vi "Connect_Netpie.vi"(6 "Subscribe":bool, 7 "Topic Subscriptions":T3[](array[typedef]), 8 "error in (no error)":errorcluster, 9 "Password":string, 10 "Username":string, 11 "ID (empty:generate new)":string="b583b29d-c581-4886-b5fe-addf69b37640") -> (0 "error out":errorcluster, 2 "Data2":string, 3 "Data1":string)   [LabVIEW 2015]
uses:
  <vilib>/LabVIEW Open Source Project/MQTT Control Packets/Control Packets/CONNECT/ConnectFlags -- cluster.ctl
  <vilib>/LabVIEW Open Source Project/MQTT Control Packets/Control Packets/SUBSCRIBE/Topic Subscription -- cluster.ctl
  <vilib>/LabVIEW Open Source Project/MQTT Control Packets/Control Packets/ControlPacket/QualityOfService -- enum.ctl
  <vilib>/LabVIEW Open Source Project/MQTT Control Packets/Control Packets/SUBACK/Subscription Success Code.ctl
  <vilib>/LabVIEW Open Source Project/MQTT Client/Client class/Client.lvclass/Client.ctl
  <vilib>/LabVIEW Open Source Project/MQTT Connection/MQTT_Base/Base Class/MQTT_Base.lvclass/MQTT_Base.ctl
  <vilib>/LabVIEW Open Source Project/MQTT Control Packets/Control Packets/ControlPacket/ControlPacket.lvclass/ControlPacket.ctl
  <vilib>/LabVIEW Open Source Project/MQTT Control Packets/Control Packets/PUBLISH/PUBLISH.lvclass
  <vilib>/LabVIEW Open Source Project/MQTT Client/Client class/Client.lvclass
  <vilib>/LabVIEW Open Source Project/MQTT Connection/MQTT_Base/Base Class/MQTT_Base.lvclass
  <vilib>/LabVIEW Open Source Project/MQTT Control Packets/Control Packets/ControlPacket/ControlPacket.lvclass
  <vilib>/LabVIEW Open Source Project/Connection/Connection.TCP/Connection.TCP.lvclass
  <vilib>/LabVIEW Open Source Project/Connection/Connection.LocalQueue/Connection.LocalQueue.lvclass
  <vilib>/LabVIEW Open Source Project/Connection/Connection/Connection.lvclass
  <vilib>/LabVIEW Open Source Project/MQTT Control Packets/Control Packets/CONNECT/CONNECT.lvclass
  <vilib>/LabVIEW Open Source Project/MQTT Control Packets/Control Packets/SUBSCRIBE/SUBSCRIBE.lvclass
  <vilib>/LabVIEW Open Source Project/MQTT Control Packets/Control Packets/SUBACK/SUBACK.lvclass
panel:
  out "error out 6":errorcluster
  out "Type 2":variant
  out "Topic 2":string
  out "error out 5":errorcluster
  out "Subscription Success":T1[](array[typedef])
  out "error out 4":errorcluster
  out "number (0 to 1)":dbl
  out "error out 3":errorcluster
  out "Topic":string
  out "Type":variant
  in  "Connect Flags":T4={"Reserved"=FALSE, "Clean Session"=TRUE, "Will Flag"=FALSE, "Will QoS 1"=FALSE, "Will QoS 2"=FALSE, "Will Retain"=FALSE, "Password Flag"=TRUE, "User Name Flag"=TRUE}
  out "error out 2":errorcluster
  in  "Payload":T5={"Will Topic"="", "Will Message"="", "Username"="ds3VmEp7KaA5nuEX2GCNHMqxBePMp4tM", "Password"="m4XKedujvHFPDgxpF4Xtp1ibe3j8miZE"}
  out "Incoming Message":u8[](array[numeric]) format="%08b"
  out "Suback":bool
  out "Published":bool
  in  "Publish":bool
  in  "Stop Client":bool
  # "ESP32_D1"
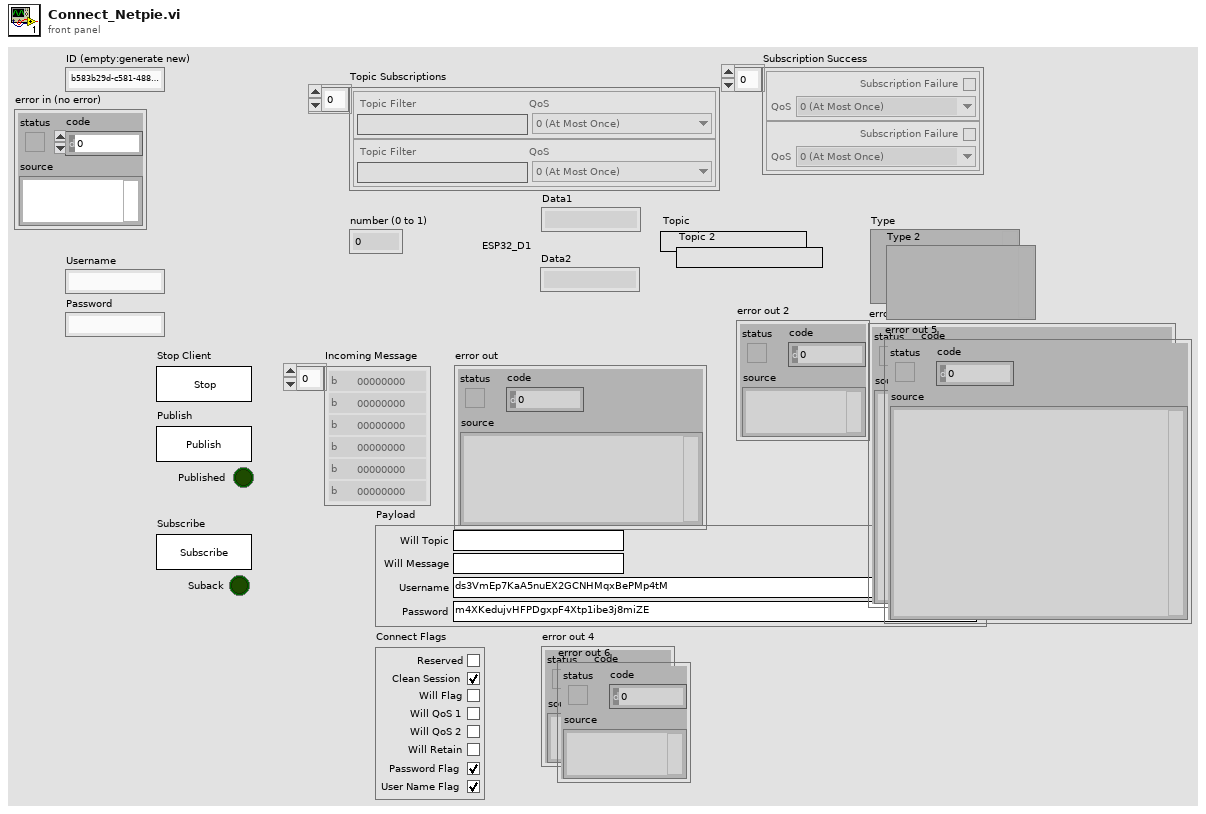
[diagram p1: front panel]
types:
  T1 = typedef "MQTT_Control_Packets.lvlib/SUBACK.lvclass/Subscription Success Code.ctl" = cluster{"Subscription Failure":bool, "QoS":T2}
  T2 = typedef "MQTT_Control_Packets.lvlib/ControlPacket.lvclass/QualityOfService -- enum.ctl" = enum16{"0 (At Most Once)", "1 (At Least Once)", "2 (Exactly Once)"}
  T3 = typedef "MQTT_Control_Packets.lvlib/SUBSCRIBE.lvclass/Topic Subscription -- cluster.ctl" = cluster{"Topic Filter":string, "QoS":T2}
  T4 = typedef "MQTT_Control_Packets.lvlib/CONNECT.lvclass/ConnectFlags -- cluster.ctl" = cluster{"Reserved":bool, "Clean Session":bool, "Will Flag":bool, "Will QoS 1":bool, "Will QoS 2":bool, "Will Retain":bool, "Password Flag":bool, "User Name Flag":bool}
  T5 = cluster{"Will Topic":string, "Will Message":string, "Username":string, "Password":string}
  T6 = typedef "MQTT Client.lvlib/Client.lvclass/Public Events -- cluster.ctl" = cluster{"Connection Status":refnum<user-event>, "Connected":refnum<user-event>, "Application Message":refnum<user-event>}
  T7 = typedef "MQTT Base.lvlib/MQTT_Base.lvclass/Public Events -- cluster.ctl" = cluster{"Stop Event":refnum<user-event>, "Error Event":refnum<user-event>, "Inbound Message":refnum<user-event>}
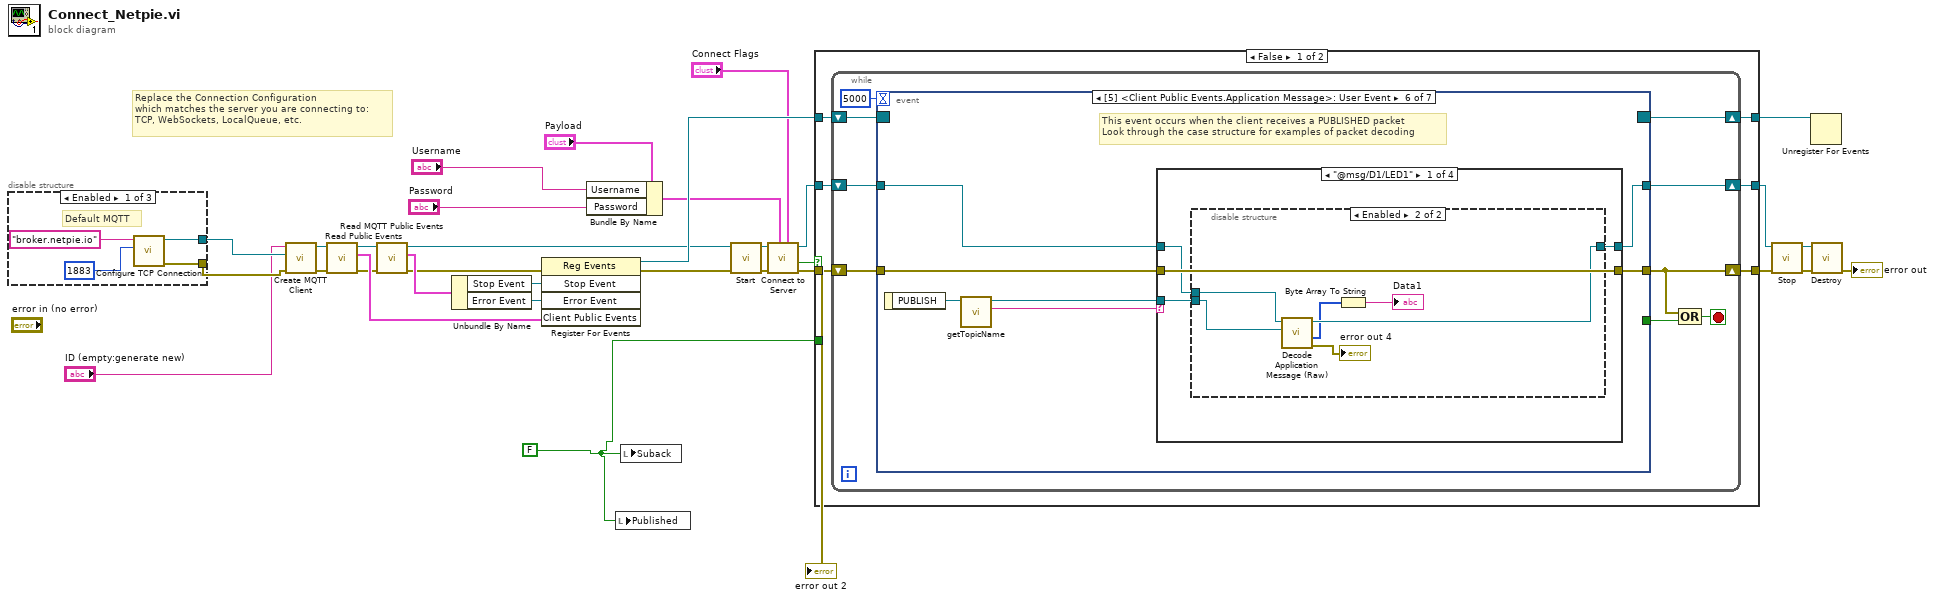
[diagram p0: block diagram]
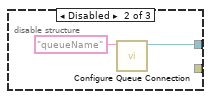
[diagram p2: hidden frame]
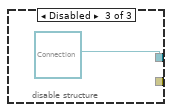
[diagram p3: hidden frame]
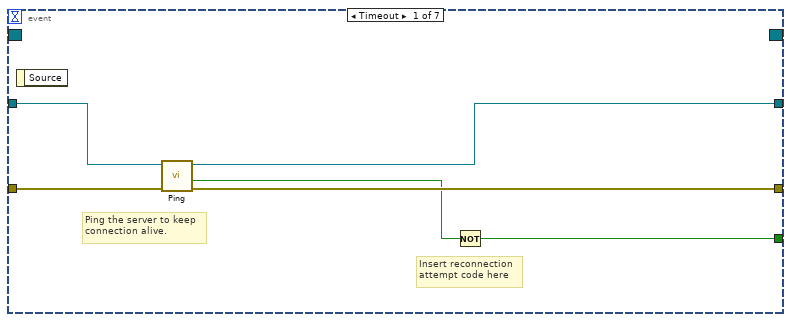
[diagram p4: hidden frame]
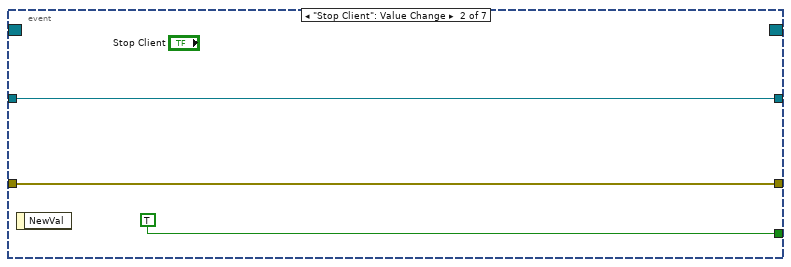
[diagram p5: hidden frame]
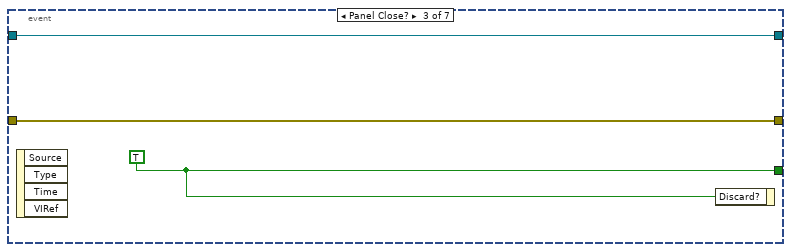
[diagram p6: hidden frame]
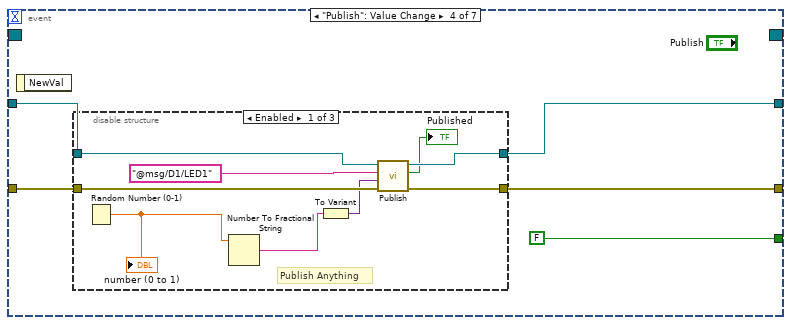
[diagram p7: hidden frame]
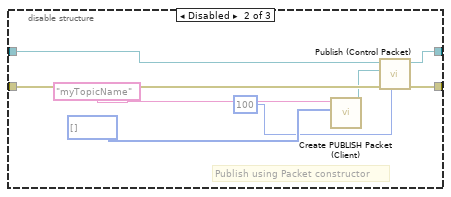
[diagram p8: hidden frame]
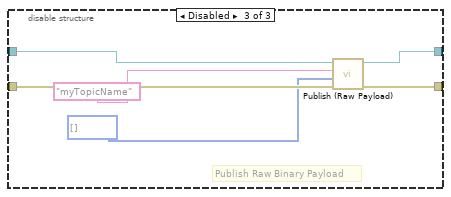
[diagram p9: hidden frame]
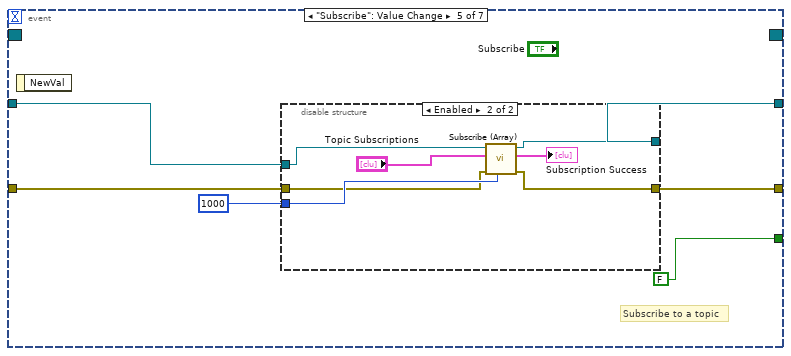
[diagram p10: hidden frame]
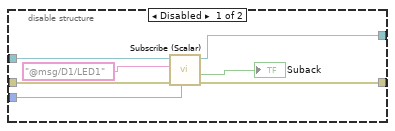
[diagram p11: hidden frame]
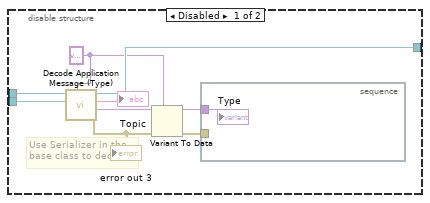
[diagram p12: hidden frame]
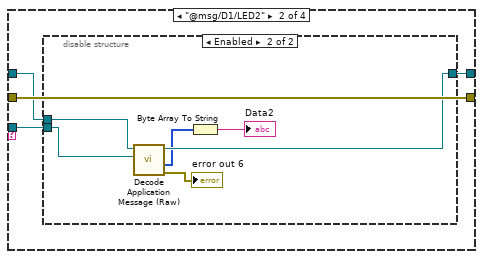
[diagram p13: hidden frame]
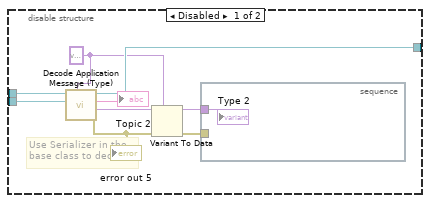
[diagram p14: hidden frame]
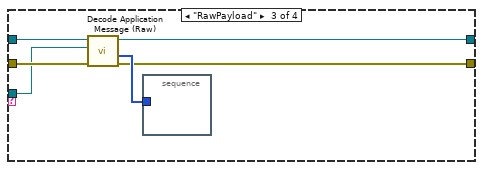
[diagram p15: hidden frame]
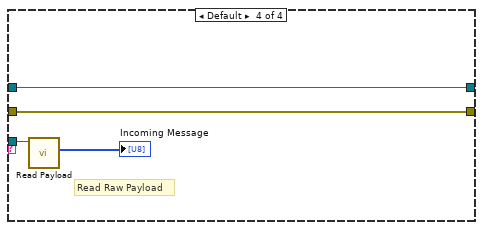
[diagram p16: hidden frame]
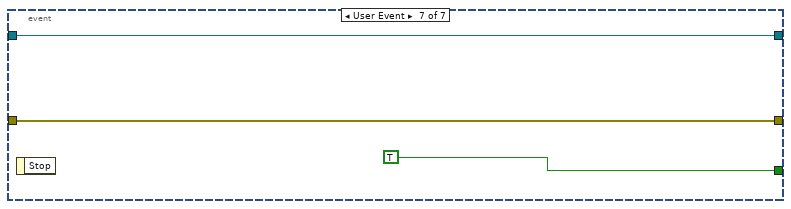
[diagram p17: hidden frame]
diagram:
  w5 = FALSE ("Suback")
  # "Replace the Connection Configuration\nwhich matches the server you are connecting to:\nTCP, WebSockets, LocalQueue, etc."
  n1 = disable-structure shown="Enabled" {
    disable-tunnel: [w35 w38 refnum<class "Connection.lvclass"> refnum ("Connection Configuration")] -> w32
    disable-tunnel: [w33 _ _] -> w8
    frame Enabled {
      # "Default MQTT"
      n2 = call <vilib>:"Configure TCP Connection.vi"("remote port (80)"=u16 1883, "address (localhost)"="broker.netpie.io") -> ("error out"=w33:errorcluster, "Connection.TCP"=w35:refnum<class "Connection.TCP.lvclass">)  [unwired: 8 in]
    }
    frame Disabled {
      n3 = call <vilib>:"Configure Queue Connection.vi"("Queue Name"="queueName") -> ("Connection.LocalQueue"=w38:refnum<class "Connection.LocalQueue.lvclass">)  [unwired: 9 in, 1 out]
    }
    frame Disabled {
    }
  }
  n4 = call <vilib>:"Create MQTT Client.vi"("error in (no error)"=w8, "Connection Configuration"=w32, "ID (empty:generate new)"="ID (empty:generate new)") -> ("error out"=w11:errorcluster, "Client out"=w9:refnum<class "Client.lvclass">)  [unwired: 7 in]
  n5 = call <vilib>:"Read Public Events.vi"("error in (no error)"=w11, "Client in"=w9) -> ("error out"=w12:errorcluster, "Client Public Events"=w14:T6, "Client out"=w10:refnum<class "Client.lvclass">)  [unwired: 7 in]
  n6 = call <vilib>:"Read MQTT Public Events.vi"("error in (no error)"=w12, "MQTT_Base in"=w10) -> ("error out"=w13:errorcluster, "MQTT Public Events"=w26:T7, "MQTT_Base out"=w16:refnum<class "Client.lvclass">)  [unwired: 7 in]
  n7 = Unbundle By Name(w26) -> ("Stop Event"=w24:refnum<user-event>, "Error Event"=w25:refnum<user-event>)
  n8 = register-events(error in=w13, w24, w25, w14) -> (reference out=w19:refnum<event-registration>, error out=w15:errorcluster)  [unwired: 1 in]
  n9 = Bundle By Name(cluster="Payload", "Username"="Username", "Password"="Password") -> (w1:T5)
  n10 = local write "Published"(w5) -> ()
  n11 = local write "Suback"(w5) -> ()
  n12 = call <vilib>:"Start.vi"("error in (no error)"=w15, "MQTT_Base in"=w16) -> ("error out"=w18:errorcluster, "MQTT_Base out"=w17:refnum<class "Client.lvclass">)  [unwired: 7 in, 1 out]
  n13 = call <vilib>:"Connect to Server.vi"("Connect Flags"="Connect Flags", "Payload"=w1, "error in (no error)"=w18, "Client in"=w17) -> ("error out"=w22:errorcluster, "timed out"=w21:bool, "Client out"=w23:refnum<class "Client.lvclass">)  [unwired: 4 in, 1 out]
  "error out 2" <- w22
  n14 = case shown="False" w21 {
    tunnel: w19 -> [w45 w177]
    tunnel: [w44 w177] -> w20
    tunnel: w22 -> [w41 w175]
    tunnel: w23 -> [w43 w176]
    tunnel: [w42 w176] -> w28
    tunnel: [w40 w175] -> w30
    tunnel: w5 -> [_ _]
    frame False {
      n15 = while {
        shift-right: [w53] -> w44
        shift-left: w45 -> [w54]
        shift-right: [w46] -> w42
        shift-left: w43 -> [w47]
        shift-right: [w51] -> w40
        shift-left: w41 -> [w52]
        stop <- w50 stop-if-true
        n16 = event shown="[5] <Client Public Events.Application Message>: User Event" {
          selector: w54 -> [_ _ _ _ _ _ _]
          dyn-events: [_ _ _ _ _ _ _] -> w53
          timeout: 5000 -> [_ _ _ _ _ _ _]
          tunnel: w52 -> [w59 w62 w64 w69 w98 w116 w174]
          tunnel: [w57 w62 w64 w68 w97 w117 w174] -> w51
          tunnel: [w56 TRUE w66 FALSE FALSE _ TRUE] -> w49
          tunnel: w47 -> [w60 w63 w65 w70 w99 w119 w172]
          tunnel: [w58 w63 w65 w67 w96 w118 w172] -> w46
          event Timeout {
            # "Insert reconnection\nattempt code here"
            # "Ping the server to keep\nconnection alive."
            n17 = event-data() -> ()  [unwired: 1 in, 1 out]
            n18 = call <vilib>:"Ping.vi"("error in (no error)"=w59, "Client in"=w60) -> ("error out"=w57:errorcluster, "Server responded"=w55:bool, "Client out"=w58:refnum<class "Client.lvclass">)  [unwired: 6 in, 1 out]
            n19 = Not(x=w55) -> (.not. x?=w56:bool)
          }
          event "Stop Client": Value Change {
            n20 = event-data() -> ()  [unwired: 1 in, 1 out]
          }
          event Panel Close? {
            w66 = TRUE
            n21 = event-data() -> ()  [unwired: 1 in, 4 out]
            n22 = event-data("Discard?"=w66) -> ()  [unwired: 1 in, 1 out]
          }
          event "Publish": Value Change {
            n23 = event-data() -> ()  [unwired: 1 in, 1 out]
            n24 = disable-structure shown="Enabled" {
              disable-tunnel: w70 -> [w80 w86 w94]
              disable-tunnel: w69 -> [w79 w84 w91]
              disable-tunnel: [w78 w83 w92] -> w68
              disable-tunnel: [w77 w85 w93] -> w67
              frame Enabled {
                # "Publish Anything"
                n25 = Random Number (0-1)() -> (number: 0 to 1=w73:dbl)
                "number (0 to 1)" <- w73
                n26 = Number To Fractional String(number=w73) -> (F-format string=w72:string)  [unwired: 3 in]
                n27 = To Variant(anything=w72) -> (Variant=w75:variant)
                n28 = call <vilib>:"Publish.vi"("error in (no error)"=w79, "Payload"=w75, "Topic Name (empty: Payload name)"="@msg/D1/LED1", "Client in"=w80) -> ("error out"=w78:errorcluster, "Published"=→"Published":bool, "Client out"=w77:refnum<class "Client.lvclass">)  [unwired: 5 in]
              }
              frame Disabled {
                # "Publish using Packet constructor"
                n29 = call <vilib>:"Create PUBLISH Packet (Client).vi"("Payload"=u8[] [], "Topic Name"="myTopicName" ("Topic Name (empty: Payload name)")) -> ("PUBLISH"=w81:refnum<class "PUBLISH.lvclass">)  [unwired: 6 in, 3 out]
                n30 = call <vilib>:"Publish (Control Packet).vi"("timeout (1000ms)"=100 ("timeout (0ms : no ack)"), "error in (no error)"=w84, "PUBLISH"=w81, "Client in"=w86) -> ("error out"=w83:errorcluster, "Client out"=w85:refnum<class "Client.lvclass">)  [unwired: 5 in, 1 out]
              }
              frame Disabled {
                # "Publish Raw Binary Payload"
                n31 = call <vilib>:"Publish (Raw Payload).vi"("error in (no error)"=w91, "Binary Payload"=u8[] [] ("Payload"), "Topic Name"="myTopicName" ("Topic Name (empty: Payload name)"), "Client in"=w94) -> ("error out"=w92:errorcluster, "Client out"=w93:refnum<class "Client.lvclass">)  [unwired: 5 in, 1 out]
              }
            }
          }
          event "Subscribe": Value Change {
            # "Subscribe to a topic"
            n32 = event-data() -> ()  [unwired: 1 in, 1 out]
            n33 = disable-structure shown="Enabled" {
              disable-tunnel: w99 -> [w107 w114]
              disable-tunnel: w98 -> [w105 w110]
              disable-tunnel: [w104 w109] -> w97
              disable-tunnel: [w103 w111] -> w96
              disable-tunnel: 1000 ("timeout (100ms)") -> [w101 w113]
              frame Disabled {
                n34 = call <vilib>:"Subscribe (Scalar).vi"("timeout (1000ms)"=w101, "error in (no error)"=w105, "Topic Filter"="@msg/D1/LED1" ("Topic Name (empty: Payload name)"), "Client in"=w107) -> ("error out"=w104:errorcluster, "Ack"=→"Suback":bool, "Client out"=w103:refnum<class "Client.lvclass">)  [unwired: 5 in]
              }
              frame Enabled {
                n35 = call <vilib>:"Subscribe (Array).vi"("timeout (1000ms)"=w113, "error in (no error)"=w110, "Topic Subscriptions"="Topic Subscriptions", "Client in"=w114) -> ("error out"=w109:errorcluster, "Subscription Success"=→"Subscription Success":T1[], "Client out"=w111:refnum<class "Client.lvclass">)  [unwired: 5 in]
              }
            }
          }
          event User Event {
            # "This event occurs when the client receives a PUBLISHED packet\nLook through the case structure for examples of packet decoding"
            n36 = event-data() -> ("PUBLISH"=w121:refnum<class "PUBLISH.lvclass">)  [unwired: 1 in]
            n37 = call <vilib>:"getTopicName.vi"("PUBLISH in"=w121) -> ("Topic"=w120:string, "PUBLISH out"=w115:refnum<class "PUBLISH.lvclass">)  [unwired: 8 in, 1 out]
            n38 = case shown="\"@msg/D1/LED1\"" w120 {
              tunnel: w119 -> [w124 w144 w167 w171]
              tunnel: [w123 w143 w166 w171] -> w118
              tunnel: [w125 w145 w164 w170] -> w117
              tunnel: w116 -> [w125 w145 w163 w170]
              tunnel: w115 -> [w122 w142 w162 w169]
              frame "@msg/D1/LED1" {
                n39 = disable-structure shown="Enabled" {
                  disable-tunnel: w124 -> [w132 w141]
                  disable-tunnel: [w131 w139] -> w123
                  disable-tunnel: w122 -> [w130 w140]
                  frame Disabled {
                    w128 = variant ("Type")
                    # "Use Serializer in the\nbase class to decode"
                    n40 = call <vilib>:"Decode Application Message (Type).vi"("Type"=w128, "PUBLISH"=w130, "Client in"=w132) -> ("error out"=w127:errorcluster, "Payload"=w129:variant, "Topic"=→"Topic":string, "Client out"=w131:refnum<class "Client.lvclass">)  [unwired: 5 in]
                    "error out 3" <- w127
                    n41 = Variant To Data(error in=w127, type=w128, Variant=w129) -> (data=w134:variant, error out=w133:errorcluster)
                    n42 = stacked-sequence {
                      tunnel: w134 -> [w135]
                      tunnel: w133 -> [_]
                      frame #0 {
                        "Type" <- w135
                      }
                    }
                  }
                  frame Enabled {
                    n43 = call <vilib>:"Decode Application Message (Raw).vi"("PUBLISH"=w140, "Client in"=w141) -> ("error out"=→"error out 4":errorcluster, "Payload"=w137:u8[], "Client out"=w139:refnum<class "Client.lvclass">)  [unwired: 6 in, 1 out]
                    n44 = Byte Array To String(unsigned byte array=w137) -> (string=→"Data1":string)
                  }
                }
              }
              frame "@msg/D1/LED2" {
                n45 = disable-structure shown="Enabled" {
                  disable-tunnel: w144 -> [w152 w161]
                  disable-tunnel: [w151 w159] -> w143
                  disable-tunnel: w142 -> [w150 w160]
                  frame Disabled {
                    w148 = variant ("Type")
                    # "Use Serializer in the\nbase class to decode"
                    n46 = call <vilib>:"Decode Application Message (Type).vi"("Type"=w148, "PUBLISH"=w150, "Client in"=w152) -> ("error out"=w147:errorcluster, "Payload"=w149:variant, "Topic"=→"Topic 2":string, "Client out"=w151:refnum<class "Client.lvclass">)  [unwired: 5 in]
                    "error out 5" <- w147
                    n47 = Variant To Data(error in=w147, type=w148, Variant=w149) -> (data=w154:variant, error out=w153:errorcluster)
                    n48 = stacked-sequence {
                      tunnel: w154 -> [w155]
                      tunnel: w153 -> [_]
                      frame #0 {
                        "Type 2" <- w155
                      }
                    }
                  }
                  frame Enabled {
                    n49 = call <vilib>:"Decode Application Message (Raw).vi"("PUBLISH"=w160, "Client in"=w161) -> ("error out"=→"error out 6":errorcluster, "Payload"=w157:u8[], "Client out"=w159:refnum<class "Client.lvclass">)  [unwired: 6 in, 1 out]
                    n50 = Byte Array To String(unsigned byte array=w157) -> (string=→"Data2":string)
                  }
                }
              }
              frame "RawPayload" {
                n51 = call <vilib>:"Decode Application Message (Raw).vi"("error in (no error)"=w163, "PUBLISH"=w162, "Client in"=w167) -> ("error out"=w164:errorcluster, "Payload"=w165:u8[], "Client out"=w166:refnum<class "Client.lvclass">)  [unwired: 5 in, 1 out]
                n52 = stacked-sequence {
                  tunnel: w165 -> [_]
                  frame #0 {
                  }
                }
              }
              frame Default {
                # "Read Raw Payload"
                n53 = call <vilib>:"Read Payload.vi"("ControlPacket in"=w169) -> ("Payload"=→"Incoming Message":u8[])  [unwired: 9 in, 1 out]
              }
            }
          }
          event User Event {
            n54 = event-data() -> ()  [unwired: 1 in, 1 out]
          }
        }
        n55 = Compound Arithmetic op=OR(w51, w49) -> (w50:bool)
      }
    }
    frame True {
    }
  }
  n56 = call <vilib>:"Stop.vi"("error in (no error)"=w30, "MQTT_Base in"=w28) -> ("error out"=w29:errorcluster, "MQTT_Base out"=w27:refnum<class "Client.lvclass">)  [unwired: 7 in, 1 out]
  n57 = Unregister For Events(event registration refnum=w20) -> ()  [unwired: 1 in, 1 out]
  n58 = call <vilib>:"Destroy.vi"("error in (no error)"=w29, "MQTT_Base in"=w27) -> ("error out"=→"error out":errorcluster)  [unwired: 8 in, 1 out]
